vi "set_Control_Array.vi"(8 "error in (no error)":errorcluster, 10 "Control Array":bool[][](array[boolean]), 11 "CtrlLine in":refnum<class "CtrlLine.lvclass">) -> (0 "error out":errorcluster, 3 "CtrlLine out":refnum<class "CtrlLine.lvclass">)   [LabVIEW 2020, in "CtrlLine.lvclass"]
uses:
  CtrlLine.lvclass
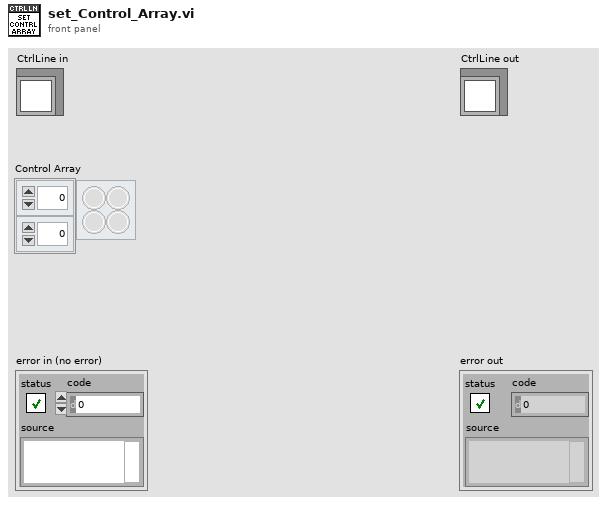
[diagram p1: front panel]
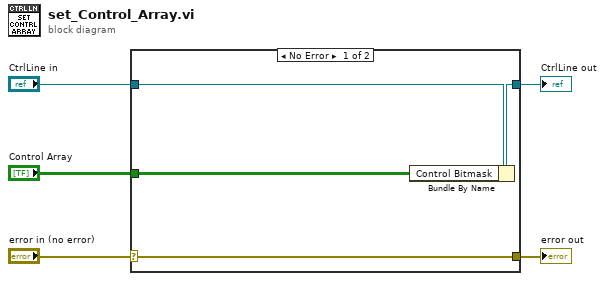
[diagram p0: block diagram]
diagram:
  n1 = case shown="No Error" "error in (no error)" {
    selector: "error in (no error)" -> [w9 w10]
    tunnel: [w9 w10] -> w4
    tunnel: [w7 w11] -> w2
    tunnel: "CtrlLine in" -> [w8 w11]
    tunnel: "Control Array" -> [w6 _]
    frame No Error {
      n2 = Bundle By Name(cluster=w8, "Control Bitmask"=w6) -> (w7:refnum<class "CtrlLine.lvclass">)
    }
    frame Error {
    }
  }
  "error out" <- w4
  "CtrlLine out" <- w2
